vi "Write Mission Controller Settings.vi"(8 "error in (no error)":errorcluster, 10 "Mission Controller Settings":T1, 11 "RDS Mission Controller Actor in":refnum<class "RDS Mission Controller Actor.lvclass">) -> (0 "error out":errorcluster, 3 "RDS Mission Controller Actor out":refnum<class "RDS Mission Controller Actor.lvclass">)   [LabVIEW 2015, in "RDS Mission Controller Actor.lvlib" / "RDS Mission Controller Actor.lvclass"]
uses:
  RDS Mission Controller Actor.lvclass
  Mission Controller Settings.ctl
  RDS Mission Controller Actor.lvclass/RDS Mission Controller Actor.ctl
  RDS Mission Controller Actor.lvlib
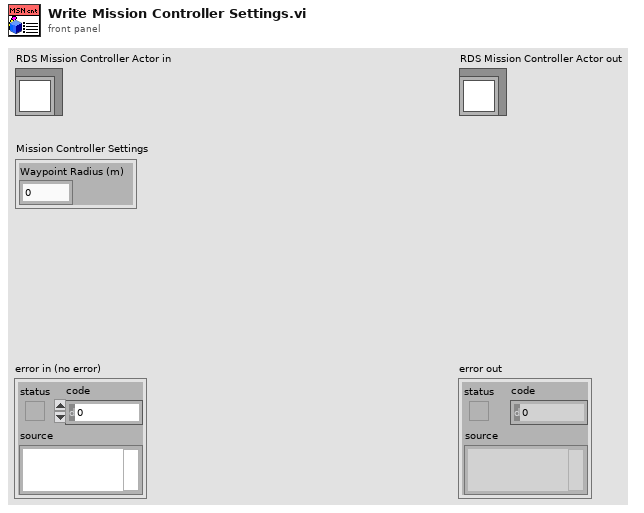
[diagram p1: front panel]
types:
  T1 = typedef "RDS Mission Controller Actor.lvlib/Mission Controller Settings.ctl" = cluster{"Waypoint Radius (m)":dbl}
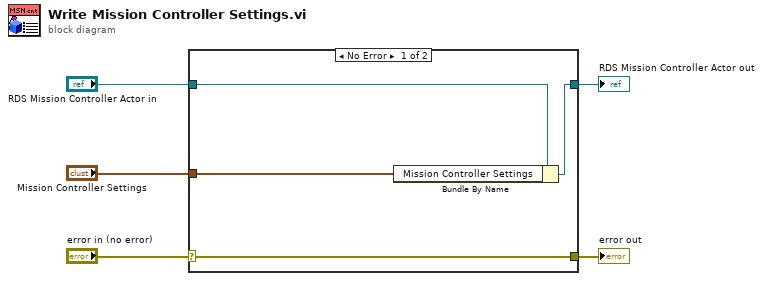
[diagram p0: block diagram]
diagram:
  n1 = case shown="No Error" "error in (no error)" {
    selector: "error in (no error)" -> [w9 w10]
    tunnel: [w9 w10] -> w4
    tunnel: [w7 w11] -> w2
    tunnel: "RDS Mission Controller Actor in" -> [w8 w11]
    tunnel: "Mission Controller Settings" -> [w6 _]
    frame No Error {
      n2 = Bundle By Name(cluster=w8, "Mission Controller Settings"=w6) -> (w7:refnum<class "RDS Mission Controller Actor.lvclass">)
    }
    frame Error {
    }
  }
  "error out" <- w4
  "RDS Mission Controller Actor out" <- w2
